vi "KLN.vi"(0 "System no.":i32=1 min=1 max=4 step=1, 2 "Child CS":string, 3 "Parent CS":string, 5 "error in":errorcluster) -> (19 "error out":errorcluster)   [LabVIEW 2026]
doc: "Links two coordinate systems together by defining a parent-child relation; thus forming a chain, and queries ERR?. \nKLN does not allow linking a coordinate system to itself. KLN does not check for cyclic coordinate system relations. Check is done with KEN. Linking a KSB-type coordinate system as child requires command level 1 (CCL.vi). Coordinate system settings are volatile but can be saved as power-on default with WPA.vi using the password \"SKS\". Controller error is TRUE if selected system reports error code not equal to 0.\n\nC-887, F-206, M-8X0: Only for GCS syntax version = GCS 2.0 or higher (Check with CSV?.vi. If CSV?.vi is not supported, syntax version is GCS 1.0)."
panel:
  # "Links two coordinate systems together by defining a parent-child relation; thus \nforming a chain,  and queries for ERR?."
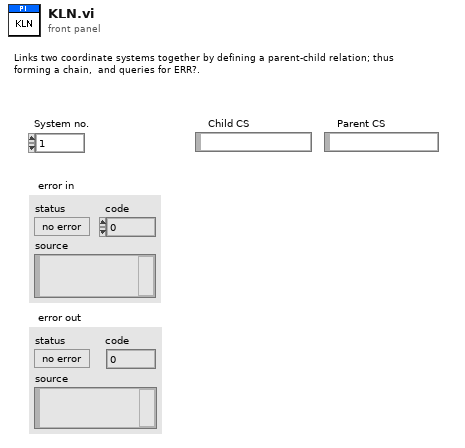
[diagram p1: front panel]
types:
  T1 = enum16{"Disable error check", "Force error check", "Use global settings"}
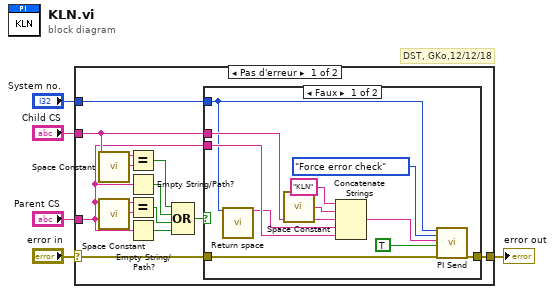
[diagram p0: block diagram]
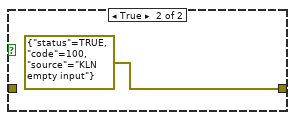
[diagram p2: hidden frame]
diagram:
  # "DST, GKo,12/12/18"
  n1 = case shown="Pas d'erreur" "error in" {
    selector: "error in" -> [w11 w30]
    tunnel: "Child CS" -> [w12 _]
    tunnel: [w10 w30] -> w5
    tunnel: "Parent CS" -> [w7 _]
    tunnel: "System no." -> [w17 _]
    frame No Error {
      n2 = call <vilib>:"Space Constant.vi"() -> ("String"=w16:string)
      n3 = call <vilib>:"Space Constant.vi"() -> ("String"=w15:string)
      n4 = Equal?(x=w12, y=w16) -> (x = y?=w14:bool)
      n5 = Empty String/Path?(string/path=w7) -> (empty?=w9:bool)
      n6 = Equal?(x=w7, y=w15) -> (x = y?=w13:bool)
      n7 = Empty String/Path?(string/path=w7) -> (empty?=w8:bool)
      n8 = Compound Arithmetic op=OR(w14, w9, w13, w8) -> (w6:bool)
      n9 = case shown="Faux" w6 {
        tunnel: w17 -> [w18 _]
        tunnel: w12 -> [w21 _]
        tunnel: w11 -> [w28 _]
        tunnel: [w27 errorcluster {"status"=TRUE, "code"=100, "source"="KLN empty input"} ("error out")] -> w10
        tunnel: w7 -> [w20 _]
        frame False {
          n10 = call "Return space.vi"("System no."=w18) -> ("String out"=w19:string)  [unwired: 1 in, 17 out]
          n11 = call <vilib>:"Space Constant.vi"() -> ("String"=w22:string)
          n12 = Concatenate Strings("KLN", w22, w21, w19, w20) -> (w24:string)
          n13 = call "PI Send.vi"("System no."=w18, "Error check settings"=T1."Force error check", "String to send"=w24, "Attach termination char.?"=TRUE ("Attach Linefeed?"), "error in"=w28) -> ("error out"=w27:errorcluster)  [unwired: 1 in, 13 out]
        }
        frame True {
        }
      }
    }
    frame Error {
    }
  }
  "error out" <- w5
